vi "GetOutputWireBranches.vi"(6 "error in":errorcluster, 9 "Node in":refnum<class "Node.lvclass">) -> (0 "error out":errorcluster, 3 "Node out":refnum<class "Node.lvclass">, 4 "branches":string[](array[string]))   [LabVIEW 2014, in "Raspberry Pi Compatible Compiler for LabVIEW.lvlib" / "Node.lvclass"]
uses:
  Node.lvclass
  Terminal/Terminal.lvclass
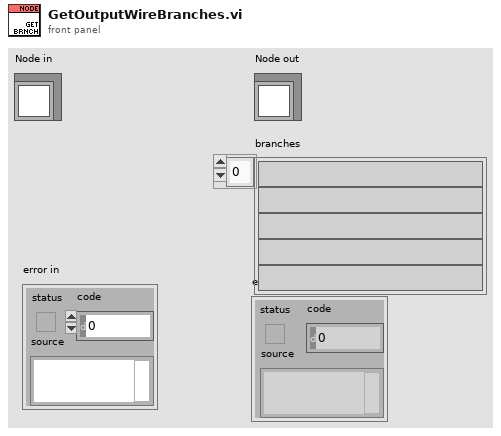
[diagram p1: front panel]
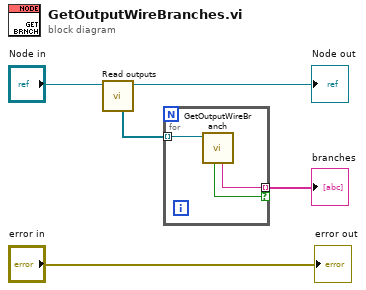
[diagram p0: block diagram]
diagram:
  n1 = call-dynamic "Read outputs.vi"("Node in"="Node in") -> ("Node out"=→"Node out":refnum<class "Node.lvclass">, "outputs"=w4:refnum<class "Terminal.lvclass">[])  [unwired: 7 in]
  n2 = for {
    tunnel: w4 -> [w8] mode=indexing
    tunnel: [w6] -> w1 mode=indexing if=w7
    n3 = call-dynamic "GetOutputWireBranch.vi"("Terminal in"=w8) -> ("branches"=w6:string, "branched"=w7:bool)  [unwired: 5 in, 2 out]
  }
  "branches" <- w1
  "error out" <- "error in"
